vi "String Functions.vi"() -> ()   [LabVIEW 2022 SP3]
panel:
  out "substring":string
  in  "String 5":string
  out "y":i32
  out "concatenated string":string
  in  "String 4":string
  in  "String 3":string
  out "Numeric":dbl
  out "String 2":string
  in  "String":string
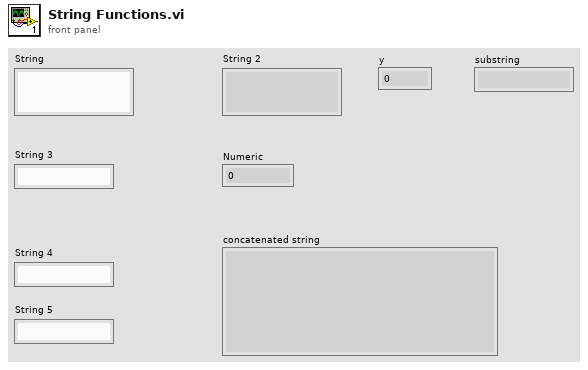
[diagram p1: front panel]
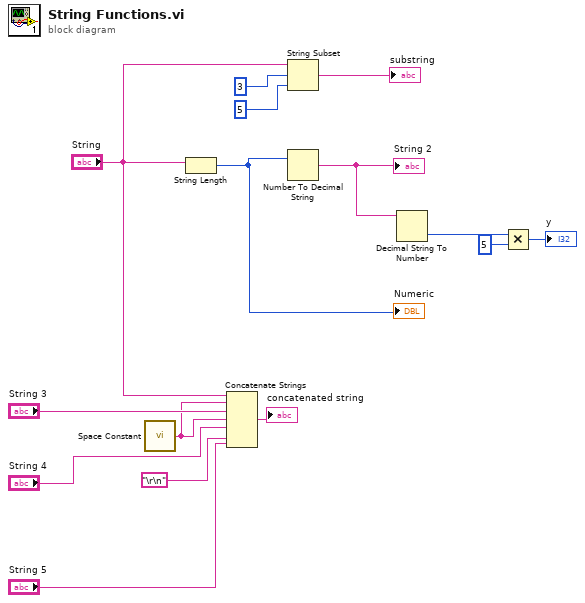
[diagram p0: block diagram]
diagram:
  n1 = call <vilib>:"Space Constant.vi"() -> ("String"=w11:string)
  n2 = String Length(string="String") -> (length=w15:i32)
  "Numeric" <- w15
  n3 = Concatenate Strings("String", w11, "String 3", w11, "String 4", "\r\n", "String 5") -> (→"concatenated string":string)
  n4 = String Subset(string="String", offset (0)=3, length (rest)=5 ("length (rest)")) -> (substring=→"substring":string)
  n5 = Number To Decimal String(number=w15) -> (decimal integer string=w14:string)  [unwired: 1 in]
  "String 2" <- w14
  n6 = Decimal String To Number(string=w14) -> (number=w13:i32)  [unwired: 2 in, 1 out]
  n7 = Multiply(x=w13, y=5) -> (x*y=→"y":i32)
